vi "_TangoSubscribeAttributeValueEvent.vi"(0 "device name":string, 1 "attribute name":string, 2 "tango event type":T1=enum."UNKNOWN_EVENT", 3 "error in":errorcluster, 4 "attribute event ref.":T2) -> (5 "evt identifier":i32, 6 "error out":errorcluster)   [LabVIEW 2014, in "tango.lvlib"]
uses:
  tango.lvlib
  _EventType.ctl
  tango_binding.so
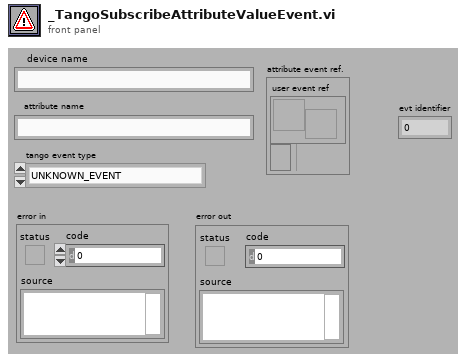
[diagram p1: front panel]
types:
  T1 = typedef "tango.lvlib/_EventType.ctl" = enum32{"CHANGE_EVENT", "DEPRECATED_QUALITY_EVENT", "PERIODIC_EVENT", "ARCHIVE_EVENT", "USER_EVENT", "ATTRIBUTE_CONF_EVENT", "DATA_READY_EVENT", "INTERFACE_CHANGE_EVENT", "UNKNOWN_EVENT"}
  T2 = cluster{"user event ref":refnum<user-event>, "user event reg refnum":refnum<event-registration>}
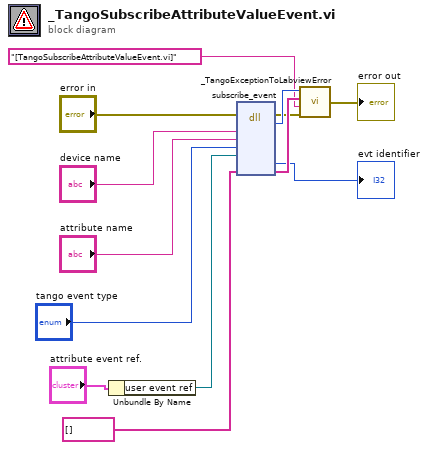
[diagram p0: block diagram]
diagram:
  n1 = Unbundle By Name("attribute event ref.") -> ("user event ref"=w3:refnum<user-event>)
  n2 = dll-call lib="tango_binding.*" fn="subscribe_event"(error in="error in", "dev_name"="device name", "attr_name"="attribute name", "evt_type"="tango event type", "evt_ref"=w3, "error_stack_"=string[] [] ("subscribe error stack")) -> (error out=w7:errorcluster, "return type"=w10:i32, "evt_identifier"=→"evt identifier":i32, "error_stack_"=w9:string[])  [unwired: 7 in, 1 out]
  n3 = call "_TangoExceptionToLabviewError.vi"("error in"=w7, "location"="[TangoSubscribeAttributeValueEvent.vi]", "error stack"=w9, "error code"=w10) -> ("error out"=→"error out":errorcluster)
